vi "TriggerTests_1_2bis.vi"() -> ()   [LabVIEW 2009]
uses:
  <vilib>/Utility/NIReport.llb/NI_report.lvclass
panel:
  out "error out 2":errorcluster
  in  "Report Enable":bool=TRUE
  in  "Curve data path":path=path "D:/CTA/IntegrationBoard/tmp"
  in  "Instrument VISA in":T1={"AWG VISA"="81160A", "Oscilloscope  VISA "="DSO80204B", "Integration Board IP"="172.16.7.43", "connection ID"=refnum, "report out"=refnum}
  out "error out":errorcluster
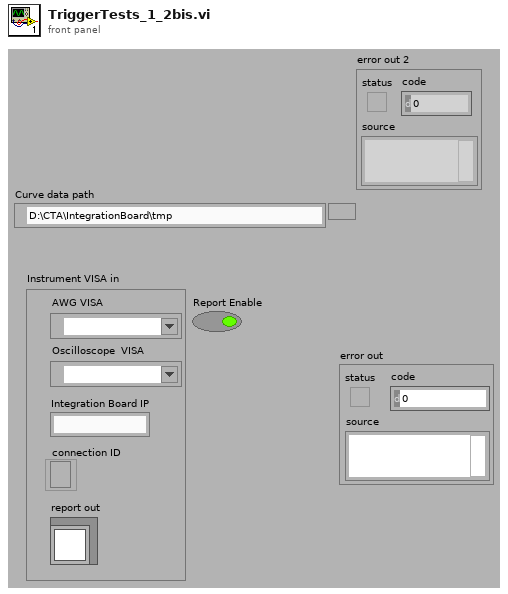
[diagram p1: front panel]
types:
  T1 = cluster{"AWG VISA":refnum<visa-resource-name>, "Oscilloscope  VISA ":refnum<visa-resource-name>, "Integration Board IP":string, "connection ID":refnum<k5>, "report out":refnum<class "NI_report.lvclass">}
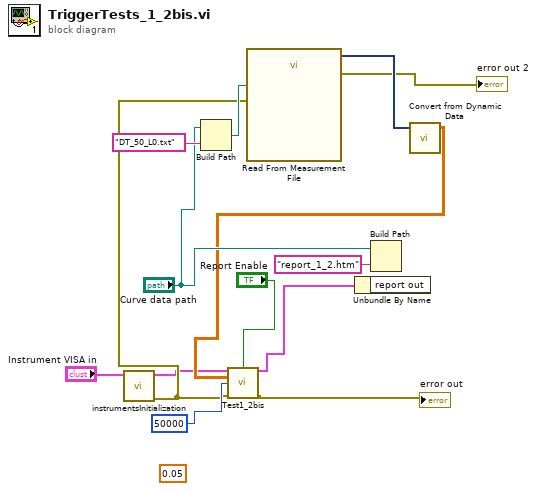
[diagram p0: block diagram]
diagram:
  (unwired) 0.05 ("Voltage Step")
  n1 = call "instrumentsInitialization.vi"("Instrument VISA in"="Instrument VISA in") -> ("error out"=w5:errorcluster, "Instrument VISA out"=w2:T1)  [unwired: 9 in]
  n2 = Build Path(base path="Curve data path", name or relative path="DT_50_L0.txt" ("Comment")) -> (appended path=w11:path)
  n3 = call "Read From Measurement File"("error in (no error)"=w5, "Filename"=w11) -> ("error out"=→"error out 2":errorcluster, "Signals"=w10:dynamicdata)  [unwired: 4 in, 4 out]
  n4 = Build Path(base path="Curve data path", name or relative path="report_1_2.htm") -> ()  [unwired: 1 out]
  n5 = call "Convert from Dynamic Data"("Dynamic Data Type"=w10) -> ("Array"=w3:dbl[][])  [unwired: 3 in]
  n6 = call "Test1_2bis.vi"("Instrument VISA in"=w2, "Report Enable"="Report Enable", "DT_50_L0"=w3, "Cycles Burst"=50000, "error in"=w5) -> ("Instrument VISA out"=w8:T1, "error out"=→"error out":errorcluster)  [unwired: 9 in]
  n7 = Unbundle By Name(w8) -> ()  [unwired: 1 out]
